vi "Untitled 3.vi"() -> ()   [LabVIEW 2011]
panel:
  out "subarray 2":i32[][](array[numeric])
  out "subarray":i32[][](array[numeric])
  out "Array":i32[][][](array[numeric])
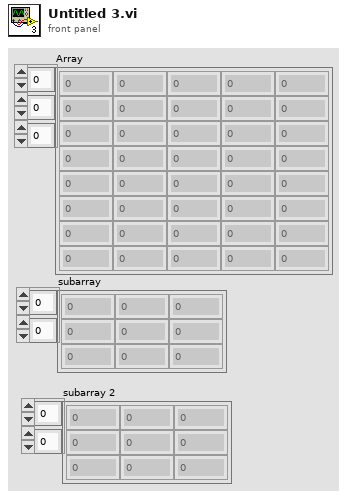
[diagram p1: front panel]
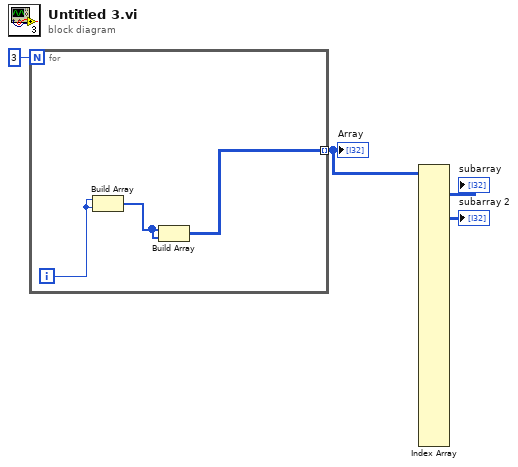
[diagram p0: block diagram]
diagram:
  n1 = for {
    N: 3 -> [_]
    tunnel: [w5] -> w3 mode=indexing
    i -> [w7]
    n2 = Build Array(w7, w7) -> (w6:i32[])
    n3 = Build Array(w6, w6) -> (w5:i32[][])
  }
  "Array" <- w3
  n4 = Index Array(array=w3) -> (element #1=→"subarray":i32[][], element #2=→"subarray 2":i32[][])  [unwired: 33 in, 9 out]
